vi "DoTeleop.vi"   [LabVIEW 2019]
uses:
  Framework/Robot Global Data.vi
  <vilib>/Rock Robotics/WPI/DriverStation/WPI_DriverStationDerivedRobotMode.ctl
types:
  T1 = typedef "WPI_DriverStationDerivedRobotMode.ctl" = enum16{"Init", "Execute", "Stop"}
  T2 = typedef "WPI_JoystickDevRef.ctl" = cluster{"Device":T3}
  T3 = typedef "WPI_JoystickDeviceEnum.ctl" = enum16{"USB 0", "USB 1", "USB 2", "USB 3", "USB 4", "USB 5"}
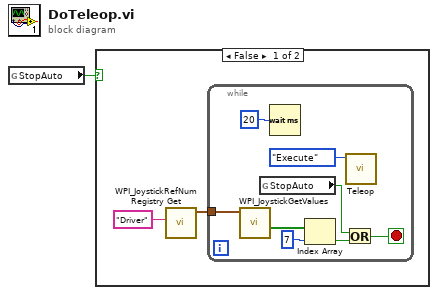
[diagram p0: block diagram]
diagram:
  n1 = global read "Robot Global Data.vi" "StopAuto"() -> (w1:bool)
  n2 = case shown="False" w1 {
    frame False {
      n3 = call <vilib>:"WPI_JoystickRefNum Registry Get.vi"("refnum name"="Driver") -> ("JoystickDevRef"=w2:T2)  [unwired: 9 in, 1 out]
      n4 = while {
        tunnel: w2 -> [w11]
        stop <- w5 stop-if-true
        n5 = call <vilib>:"WPI_JoystickGetValues.vi"("JoystickDevRef"=w11) -> ("Buttons"=w9:bool[])  [unwired: 6 in, 4 out]
        n6 = global read "Robot Global Data.vi" "StopAuto"() -> (w6:bool)
        n7 = Wait (ms)(milliseconds to wait=u32 20) -> ()  [unwired: 1 out]
        n8 = Index Array(array=w9, index=7) -> (element=w7:bool)
        n9 = Or(x=w6, y=w7) -> (x .or. y?=w5:bool)
        n10 = call "Teleop.vi"("Call Context"=WPI_DriverStationDerivedRobotMode."Execute") -> ()  [unwired: 11 in]
      }
    }
    frame True {
    }
  }
